vi "Merge.vi"(8 "error in (no error)":errorcluster, 10 "JSONText":string, 11 "BaselineDTO":T1={"schemaVersion"="", "globalThreshold"="INFO", "defaultFileAppender"={"common"={"id"="", "threshold"="INFO", "filter"={"mode"="mirror", "levelMin"="INFO", "levelMax"="INFO", "tagPrefix"=""}, "queueBound"=-1, "dropPolicy"="dropOldest", "useUTC"=FALSE}, "file"={"rootFolder"="", "maxFileSize"=-1, "maxFileCount"=-1, "baseName"="", "extension"="", "delimiter"="", "calendarFolderTree"=FALSE}}}) -> (0 "error out":errorcluster, 3 "MergedDTO":T1={"schemaVersion"="", "globalThreshold"="INFO", "defaultFileAppender"={"common"={"id"="", "threshold"="INFO", "filter"={"mode"="mirror", "levelMin"="INFO", "levelMax"="INFO", "tagPrefix"=""}, "queueBound"=-1, "dropPolicy"="dropOldest", "useUTC"=FALSE}, "file"={"rootFolder"="", "maxFileSize"=-1, "maxFileCount"=-1, "baseName"="", "extension"="", "delimiter"="", "calendarFolderTree"=FALSE}}})   [LabVIEW 2026, in "Lumberjack.lvlib"]
doc: "Pure config merge on the string DTO. Overlay a JSON document onto a baseline LumberjackConfigDTO via Unflatten From JSON with the baseline as the default value, so keys absent from the JSON keep their baseline values (per-key override, SRS-LMBR-046). Empty JSONText passes the baseline through unchanged. No I/O; deterministic.\n\nBaseline DTO + JSON text -> merged DTO (absent keys keep baseline values)."
uses:
  Lumberjack.lvlib
  TypeDefs/ConfigDTO/LumberjackConfigDTO.ctl
  TypeDefs/ConfigDTO/FileAppenderConfigDTO.ctl
  TypeDefs/ConfigDTO/AppenderConfigDTO.ctl
  TypeDefs/ConfigDTO/FilterDTO.ctl
  TypeDefs/ConfigDTO/FileConfigDTO.ctl
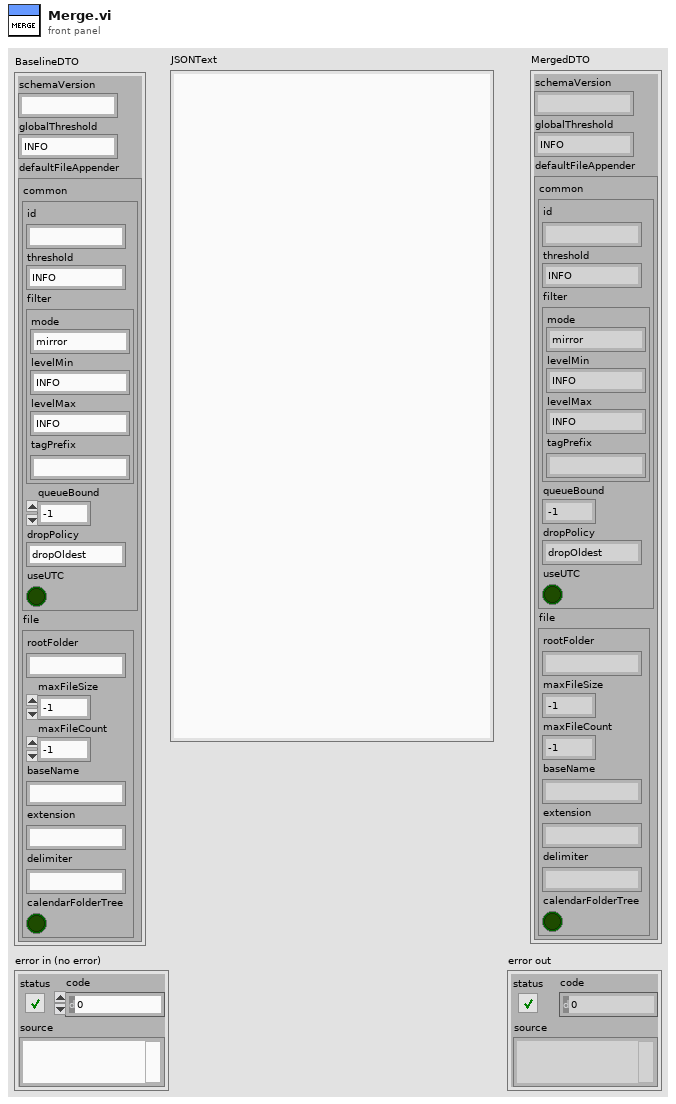
[diagram p1: front panel]
types:
  T1 = typedef "Lumberjack.lvlib/LumberjackConfigDTO.ctl" = cluster{"schemaVersion":string, "globalThreshold":string, "defaultFileAppender":T2}
  T2 = typedef "Lumberjack.lvlib/FileAppenderConfigDTO.ctl" = cluster{"common":T3, "file":T5}
  T3 = typedef "Lumberjack.lvlib/AppenderConfigDTO.ctl" = cluster{"id":string, "threshold":string, "filter":T4, "queueBound":i32, "dropPolicy":string, "useUTC":bool}
  T4 = typedef "Lumberjack.lvlib/FilterDTO.ctl" = cluster{"mode":string, "levelMin":string, "levelMax":string, "tagPrefix":string}
  T5 = typedef "Lumberjack.lvlib/FileConfigDTO.ctl" = cluster{"rootFolder":string, "maxFileSize":i64, "maxFileCount":i32, "baseName":string, "extension":string, "delimiter":string, "calendarFolderTree":bool}
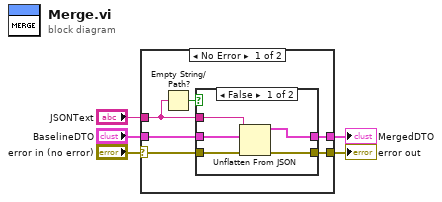
[diagram p0: block diagram]
diagram:
  n1 = case shown="No Error" "error in (no error)" {
    selector: "error in (no error)" -> [w10 w19]
    tunnel: "JSONText" -> [w7 _]
    tunnel: "BaselineDTO" -> [w11 w20]
    tunnel: [w9 w19] -> w2
    tunnel: [w8 w20] -> w1
    frame No Error {
      n2 = Empty String/Path?(string/path=w7) -> (empty?=w6:bool)
      n3 = case shown="False" w6 {
        tunnel: w7 -> [w16 _]
        tunnel: w11 -> [w15 w18]
        tunnel: w10 -> [w14 w17]
        tunnel: [w13 w17] -> w9
        tunnel: [w12 w18] -> w8
        frame False {
          n4 = Unflatten From JSON(JSON string=w16, type and defaults=w15, error in (no error)=w14) -> (value=w12:T1, error out=w13:errorcluster)  [unwired: 4 in]
        }
        frame True {
        }
      }
    }
    frame Error {
    }
  }
  "error out" <- w2
  "MergedDTO" <- w1
